vi "Date Time Channel Global.vi"() -> ()   [LabVIEW 2023]
panel:
  in  "Format Parameter Name":string="Date time format string"
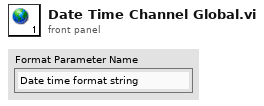
[diagram p1: front panel]
diagram:
